vi "myRIO v1.0 Build Bitmask DIO.vi"(10 "bool Value List In":bool[](array[boolean]), 11 "Channel List":T3) -> (1 "Bitmask to Channel Array":T1[](array[typedef]), 2 "OUT Bitmask Array":bool[][](array[boolean]), 3 "DIR Bitmask Array":bool[][](array[boolean]))   [LabVIEW 2021]
uses:
  <vilib>/myRIO/Common/Instrument Driver Framework/myRIO v1.0/DIO/typedefs/DIO Channels List.ctl
  <vilib>/myRIO/Common/Instrument Driver Framework/myRIO v1.0/DIO/typedefs/DIO Channels Enum.ctl
  <vilib>/myRIO/Common/Instrument Driver Framework/myRIO v1.0/DIO/typedefs/DIO Bitmask to Channel Map.ctl
  <vilib>/myRIO/Common/Instrument Driver Framework/myRIO v1.0/DIO/typedefs/DIO Bank Enum.ctl
panel:
  # "This VI is used by both the myRIO v1.0 Read DIO and Write DIO VIs. \nIf a bool Value List in is provided the appropriate OUT Botmask Array will be generated, otherwise all values in the array will be false."
  # "*Only Used for DIO Write"
  # "*Only Used for DIO Write"
  # "*Only Used for DIO Read"
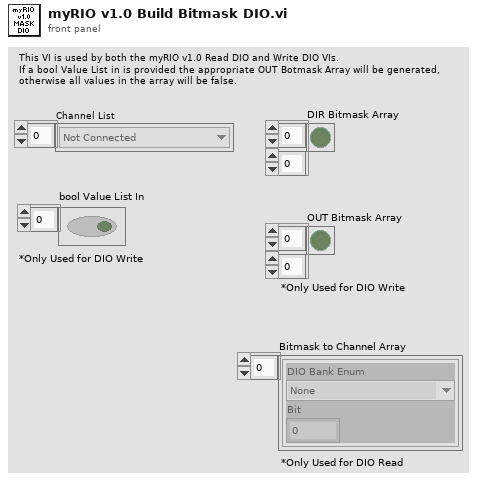
[diagram p1: front panel]
types:
  T1 = typedef "DIO Bitmask to Channel Map.ctl" = cluster{"DIO Bank Enum":T2, "Bit":i32}
  T2 = typedef "DIO Bank Enum.ctl" = enum32{"None", "C/DIO7:0", "A/DIO7:0", "A/DIO15:8", "B/DIO7:0", "B/DIO15:8", "LED3:0", "Button0"}
  T3 = typedef "DIO Channels List.ctl" = T4[]
  T4 = typedef "DIO Channels Enum.ctl" = enum16{"Not Connected", "C/DIO0", "C/DIO1", "C/DIO2", "C/DIO3", "C/DIO4", "C/DIO5", "C/DIO6", "C/DIO7", "A/DIO0", "A/DIO1", "A/DIO2", "A/DIO3", "A/DIO4", "A/DIO5", "A/DIO6", "A/DIO7", "A/DIO8", "A/DIO9", "A/DIO10", "A/DIO11", "A/DIO12", "A/DIO13", "A/DIO14", "A/DIO15", "A/DIO16", "A/DIO17", "A/DIO18", "A/DIO19", "B/DIO0", "B/DIO1", "B/DIO2", "B/DIO3", "B/DIO4", "B/DIO5", "B/DIO6", "B/DIO7", "B/DIO8", "B/DIO9", "B/DIO10", "B/DIO11", "B/DIO12", "B/DIO13", "B/DIO14", "B/DIO15", "B/DIO16", "B/DIO17", "B/DIO18", "B/DIO19", "LED0", "LED1", "LED2", "LED3", "Button0", "DIO/DIO0", "DIO/DIO1", "DIO/DIO2", "DIO/DIO3", "DIO/DIO4", "DIO/DIO5", "DIO/DIO6", "DIO/DIO7", "DIO/DIO8", "DIO/DIO9", "SPI/CS0", "SPI/CS1", "SPI/CS2", "SPI/CS3", "LED RADIO (Green)", "LED RADIO (Red)", "LED COMM (Green)", "LED COMM (Red)", "LED MODE (Green)", "LED MODE (Red)"}
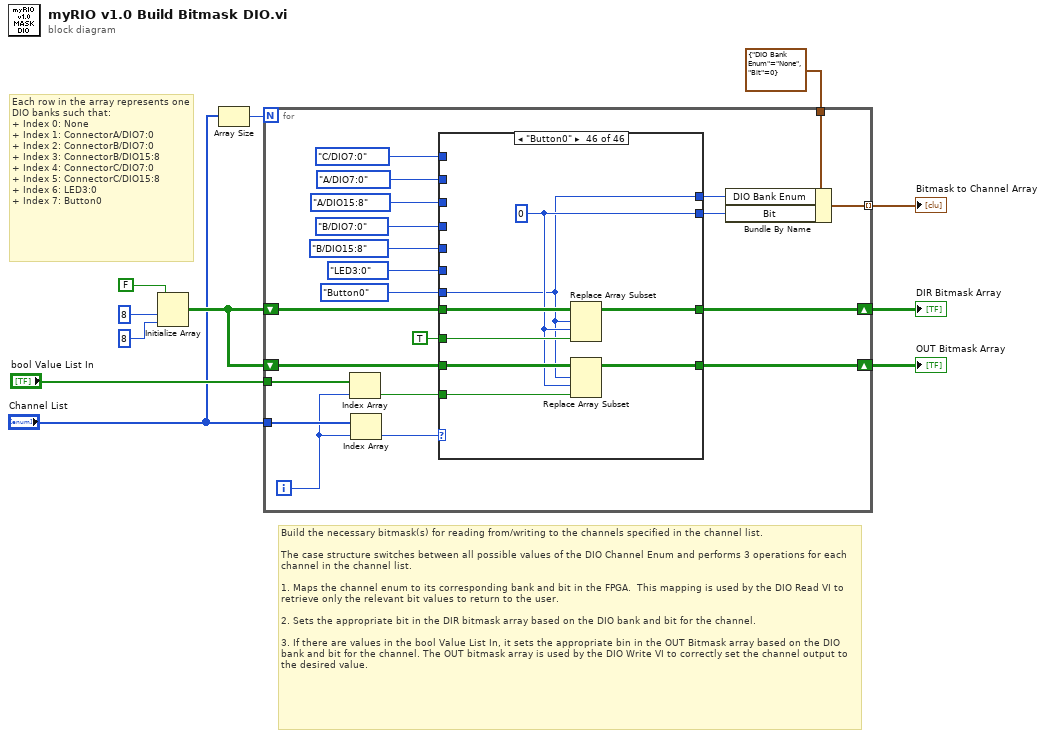
[diagram p0: block diagram]
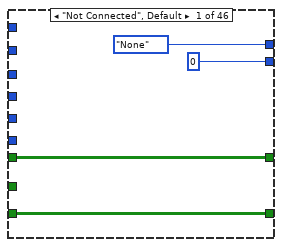
[diagram p2: hidden frame]
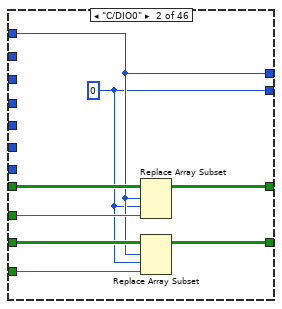
[diagram p3: hidden frame]
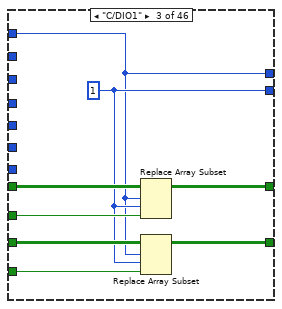
[diagram p4: hidden frame]
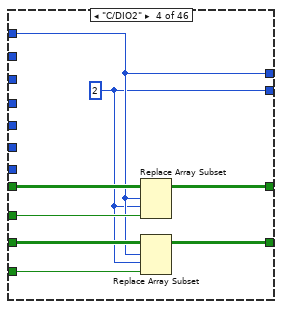
[diagram p5: hidden frame]
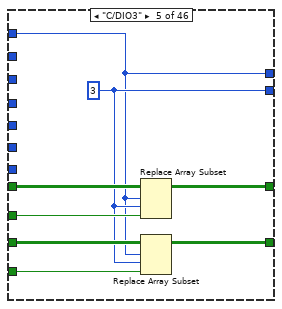
[diagram p6: hidden frame]
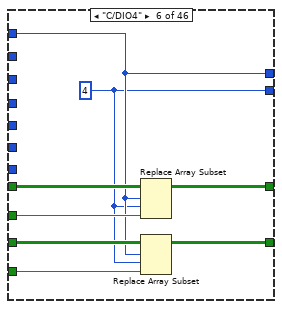
[diagram p7: hidden frame]
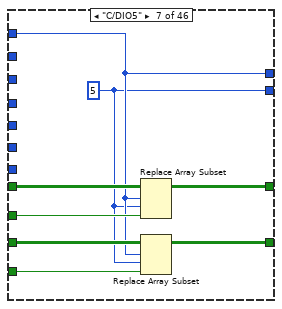
[diagram p8: hidden frame]
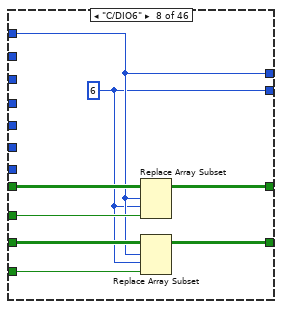
[diagram p9: hidden frame]
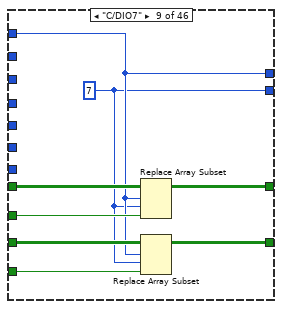
[diagram p10: hidden frame]
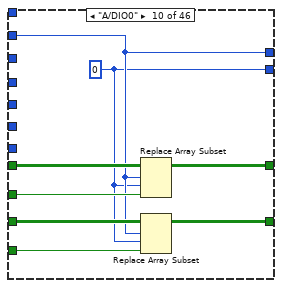
[diagram p11: hidden frame]
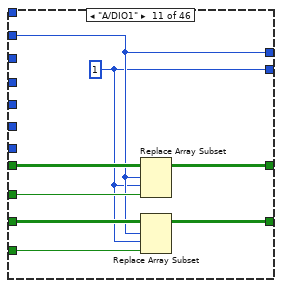
[diagram p12: hidden frame]
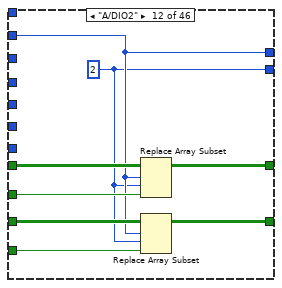
[diagram p13: hidden frame]
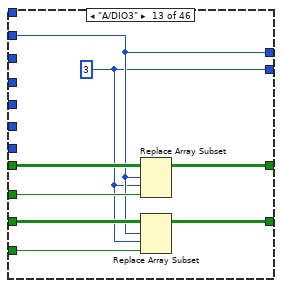
[diagram p14: hidden frame]
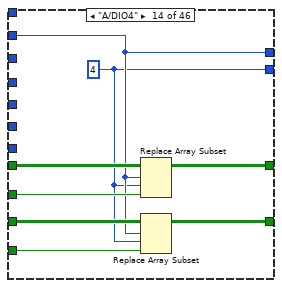
[diagram p15: hidden frame]
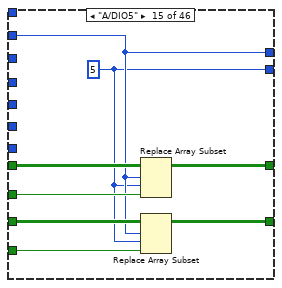
[diagram p16: hidden frame]
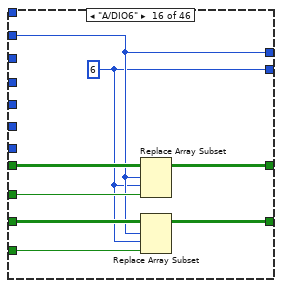
[diagram p17: hidden frame]
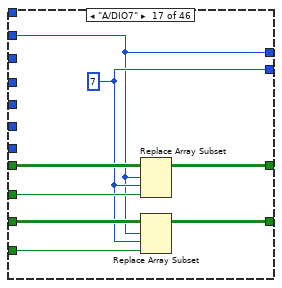
[diagram p18: hidden frame]
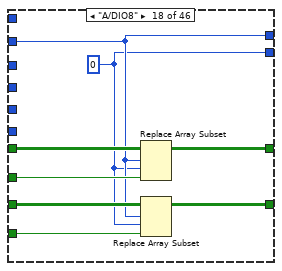
[diagram p19: hidden frame]
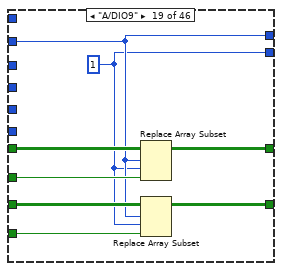
[diagram p20: hidden frame]
diagram:
  # "Build the necessary bitmask(s) for reading from/writing to the channels specified in the channel list.\n\nThe case structure switches between all possible values of the DIO Channel Enum and performs 3 operations for each channel in the channel list. \n\n1. Maps the channel enum to its corresponding bank and bit in the FPGA.  This mapping is used by the DIO Read VI to retrieve only the relevant bit values to return to the user.\n\n2. Sets the appropriate bit in the DIR bitmask array based on the DIO bank and bit for the channel.\n\n3. If there are values in the bool Value List In, it sets the appropriate bin in the OUT Bitmask array based on the DIO bank and bit for the channel. The OUT bitmask array is used by the DIO Write VI to correctly set the channel output to the desired value."
  # "Each row in the array represents one DIO banks such that:\n+ Index 0: None\n+ Index 1: ConnectorA/DIO7:0\n+ Index 2: ConnectorB/DIO7:0\n+ Index 3: ConnectorB/DIO15:8\n+ Index 4: ConnectorC/DIO7:0\n+ Index 5: ConnectorC/DIO15:8\n+ Index 6: LED3:0\n+ Index 7: Button0"
  n1 = Initialize Array(FALSE, 8 ("dimension size"), 8 ("dimension size")) -> (w5:bool[][])
  n2 = Array Size(array="Channel List") -> (size(s)=w2:i32)
  n3 = for {
    N: w2 -> [_]
    tunnel: "Channel List" -> [w17]
    shift-right: [w30] -> w10
    shift-left: w5 -> [w32]
    tunnel: T1 {"DIO Bank Enum"=enum."None", "Bit"=0} -> [w29]
    tunnel: [w27] -> w6 mode=indexing
    shift-right: [w19] -> w4
    shift-left: w5 -> [w20]
    tunnel: "bool Value List In" -> [w18]
    i -> [w15]
    n4 = Index Array(array=w18, index=w15) -> (element=w14:bool)
    n5 = Index Array(array=w17, index=w15) -> (element=w16:T4)
    n6 = case shown="\"Button0\"" w16 {
      tunnel: w32 -> [w36 w44 w52 w60 w68 w76 w84 w92 w100 w108 w116 w124 w132 w140 w148 w156 w164 w172 w180 w188 w196 w204 w212 w220 w228 w236 w244 w252 w260 w268 w276 w284 w292 w300 w308 w316 w324 w332 w340 w348 w356 w364 w372 w380 w388 w396]
      tunnel: TRUE ("new element/subarray") -> [_ w42 w50 w59 w67 w74 w82 w90 w99 w107 w114 w123 w130 w138 w146 w154 w162 w170 w178 w186 w194 w202 w210 w218 w226 w234 w242 w250 w258 w266 w274 w282 w290 w298 w306 w314 w322 w330 w338 w346 w355 w363 w371 w379 w387 w395]
      tunnel: [w36 w43 w51 w58 w66 w75 w83 w91 w98 w106 w115 w121 w131 w139 w147 w155 w163 w171 w179 w187 w195 w203 w211 w219 w227 w235 w243 w251 w259 w267 w275 w283 w291 w299 w307 w315 w323 w331 w339 w347 w354 w362 w370 w378 w386 w394] -> w30
      tunnel: [0 ("disabled index (col)") w38 w47 w54 w63 w70 w78 w86 w94 w102 w110 w118 w125 w134 w142 w150 w159 w166 w174 w182 w190 w198 w206 w214 w222 w231 w239 w247 w255 w263 w271 w279 w287 w295 w303 w311 w319 w327 w335 w343 w350 w359 w367 w375 w383 w391] -> w28
      tunnel: [DIO_Bank_Enum."None" ("DIO Bank Enum") w39 w46 w55 w62 w71 w79 w87 w95 w103 w111 w119 w126 w135 w143 w151 w157 w167 w175 w183 w191 w199 w207 w215 w223 w229 w237 w245 w253 w261 w269 w277 w285 w293 w301 w309 w317 w325 w333 w341 w351 w357 w365 w373 w381 w389] -> w25
      tunnel: DIO_Bank_Enum."C/DIO7:0" ("DIO Bank Enum") -> [_ w39 w46 w55 w62 w71 w79 w87 w95 _ _ _ _ _ _ _ _ _ _ _ _ _ _ _ _ _ _ _ _ _ _ _ _ _ _ _ _ _ _ _ _ _ _ _ _ _]
      tunnel: DIO_Bank_Enum."A/DIO7:0" ("DIO Bank Enum") -> [_ _ _ _ _ _ _ _ _ w103 w111 w119 w126 w135 w143 w151 w157 _ _ _ _ _ _ _ _ _ _ _ _ _ _ _ _ _ _ _ _ _ _ _ _ _ _ _ _ _]
      tunnel: DIO_Bank_Enum."A/DIO15:8" ("DIO Bank Enum") -> [_ _ _ _ _ _ _ _ _ _ _ _ _ _ _ _ _ w167 w175 w183 w191 w199 w207 w215 w223 _ _ _ _ _ _ _ _ _ _ _ _ _ _ _ _ _ _ _ _ _]
      tunnel: DIO_Bank_Enum."B/DIO7:0" ("DIO Bank Enum") -> [_ _ _ _ _ _ _ _ _ _ _ _ _ _ _ _ _ _ _ _ _ _ _ _ _ w229 w237 w245 w253 w261 w269 w277 w285 _ _ _ _ _ _ _ _ _ _ _ _ _]
      tunnel: DIO_Bank_Enum."B/DIO15:8" ("DIO Bank Enum") -> [_ _ _ _ _ _ _ _ _ _ _ _ _ _ _ _ _ _ _ _ _ _ _ _ _ _ _ _ _ _ _ _ _ w293 w301 w309 w317 w325 w333 w341 w351 _ _ _ _ _]
      tunnel: w20 -> [w33 w41 w49 w57 w65 w73 w81 w89 w97 w104 w112 w122 w129 w137 w144 w152 w160 w168 w176 w184 w192 w200 w208 w216 w224 w232 w240 w248 w256 w264 w272 w280 w288 w296 w304 w312 w320 w328 w336 w344 w353 w361 w369 w377 w385 w393]
      tunnel: [w33 w40 w48 w56 w64 w72 w80 w88 w96 w105 w113 w120 w128 w136 w145 w153 w161 w169 w177 w185 w193 w201 w209 w217 w225 w233 w241 w249 w257 w265 w273 w281 w289 w297 w305 w313 w321 w329 w337 w345 w352 w360 w368 w376 w384 w392] -> w19
      tunnel: w14 -> [_ w37 w45 w53 w61 w69 w77 w85 w93 w101 w109 w117 w127 w133 w141 w149 w158 w165 w173 w181 w189 w197 w205 w213 w221 w230 w238 w246 w254 w262 w270 w278 w286 w294 w302 w310 w318 w326 w334 w342 w349 w358 w366 w374 w382 w390]
      tunnel: DIO_Bank_Enum."LED3:0" ("DIO Bank Enum") -> [_ _ _ _ _ _ _ _ _ _ _ _ _ _ _ _ _ _ _ _ _ _ _ _ _ _ _ _ _ _ _ _ _ _ _ _ _ _ _ _ _ w357 w365 w373 w381 _]
      tunnel: DIO_Bank_Enum."Button0" ("DIO Bank Enum") -> [_ _ _ _ _ _ _ _ _ _ _ _ _ _ _ _ _ _ _ _ _ _ _ _ _ _ _ _ _ _ _ _ _ _ _ _ _ _ _ _ _ _ _ _ _ w389]
      frame "Not Connected", Default {
      }
      frame "C/DIO0" {
        w38 = 0 ("disabled index (col)")
        n7 = Replace Array Subset(array=w44, new element=w42, index (row)=w39, index (col)=w38) -> (w43:bool[][])
        n8 = Replace Array Subset(array=w41, new element=w37, index (row)=w39, index (col)=w38) -> (w40:bool[][])
      }
      frame "C/DIO1" {
        w47 = 1 ("disabled index (col)")
        n9 = Replace Array Subset(array=w52, new element=w50, index (row)=w46, index (col)=w47) -> (w51:bool[][])
        n10 = Replace Array Subset(array=w49, new element=w45, index (row)=w46, index (col)=w47) -> (w48:bool[][])
      }
      frame "C/DIO2" {
        w54 = 2 ("disabled index (col)")
        n11 = Replace Array Subset(array=w60, new element=w59, index (row)=w55, index (col)=w54) -> (w58:bool[][])
        n12 = Replace Array Subset(array=w57, new element=w53, index (row)=w55, index (col)=w54) -> (w56:bool[][])
      }
      frame "C/DIO3" {
        w63 = 3 ("disabled index (col)")
        n13 = Replace Array Subset(array=w68, new element=w67, index (row)=w62, index (col)=w63) -> (w66:bool[][])
        n14 = Replace Array Subset(array=w65, new element=w61, index (row)=w62, index (col)=w63) -> (w64:bool[][])
      }
      frame "C/DIO4" {
        w70 = 4 ("disabled index (col)")
        n15 = Replace Array Subset(array=w76, new element=w74, index (row)=w71, index (col)=w70) -> (w75:bool[][])
        n16 = Replace Array Subset(array=w73, new element=w69, index (row)=w71, index (col)=w70) -> (w72:bool[][])
      }
      frame "C/DIO5" {
        w78 = 5 ("disabled index (col)")
        n17 = Replace Array Subset(array=w84, new element=w82, index (row)=w79, index (col)=w78) -> (w83:bool[][])
        n18 = Replace Array Subset(array=w81, new element=w77, index (row)=w79, index (col)=w78) -> (w80:bool[][])
      }
      frame "C/DIO6" {
        w86 = 6 ("disabled index (col)")
        n19 = Replace Array Subset(array=w92, new element=w90, index (row)=w87, index (col)=w86) -> (w91:bool[][])
        n20 = Replace Array Subset(array=w89, new element=w85, index (row)=w87, index (col)=w86) -> (w88:bool[][])
      }
      frame "C/DIO7" {
        w94 = 7 ("disabled index (col)")
        n21 = Replace Array Subset(array=w100, new element=w99, index (row)=w95, index (col)=w94) -> (w98:bool[][])
        n22 = Replace Array Subset(array=w97, new element=w93, index (row)=w95, index (col)=w94) -> (w96:bool[][])
      }
      frame "A/DIO0" {
        w102 = 0 ("disabled index (col)")
        n23 = Replace Array Subset(array=w108, new element=w107, index (row)=w103, index (col)=w102) -> (w106:bool[][])
        n24 = Replace Array Subset(array=w104, new element=w101, index (row)=w103, index (col)=w102) -> (w105:bool[][])
      }
      frame "A/DIO1" {
        w110 = 1 ("disabled index (col)")
        n25 = Replace Array Subset(array=w116, new element=w114, index (row)=w111, index (col)=w110) -> (w115:bool[][])
        n26 = Replace Array Subset(array=w112, new element=w109, index (row)=w111, index (col)=w110) -> (w113:bool[][])
      }
      frame "A/DIO2" {
        w118 = 2 ("disabled index (col)")
        n27 = Replace Array Subset(array=w124, new element=w123, index (row)=w119, index (col)=w118) -> (w121:bool[][])
        n28 = Replace Array Subset(array=w122, new element=w117, index (row)=w119, index (col)=w118) -> (w120:bool[][])
      }
      frame "A/DIO3" {
        w125 = 3 ("disabled index (col)")
        n29 = Replace Array Subset(array=w132, new element=w130, index (row)=w126, index (col)=w125) -> (w131:bool[][])
        n30 = Replace Array Subset(array=w129, new element=w127, index (row)=w126, index (col)=w125) -> (w128:bool[][])
      }
      frame "A/DIO4" {
        w134 = 4 ("disabled index (col)")
        n31 = Replace Array Subset(array=w140, new element=w138, index (row)=w135, index (col)=w134) -> (w139:bool[][])
        n32 = Replace Array Subset(array=w137, new element=w133, index (row)=w135, index (col)=w134) -> (w136:bool[][])
      }
      frame "A/DIO5" {
        w142 = 5 ("disabled index (col)")
        n33 = Replace Array Subset(array=w148, new element=w146, index (row)=w143, index (col)=w142) -> (w147:bool[][])
        n34 = Replace Array Subset(array=w144, new element=w141, index (row)=w143, index (col)=w142) -> (w145:bool[][])
      }
      frame "A/DIO6" {
        w150 = 6 ("disabled index (col)")
        n35 = Replace Array Subset(array=w156, new element=w154, index (row)=w151, index (col)=w150) -> (w155:bool[][])
        n36 = Replace Array Subset(array=w152, new element=w149, index (row)=w151, index (col)=w150) -> (w153:bool[][])
      }
      frame "A/DIO7" {
        w159 = 7 ("disabled index (col)")
        n37 = Replace Array Subset(array=w164, new element=w162, index (row)=w157, index (col)=w159) -> (w163:bool[][])
        n38 = Replace Array Subset(array=w160, new element=w158, index (row)=w157, index (col)=w159) -> (w161:bool[][])
      }
      frame "A/DIO8" {
        w166 = 0 ("disabled index (col)")
        n39 = Replace Array Subset(array=w172, new element=w170, index (row)=w167, index (col)=w166) -> (w171:bool[][])
        n40 = Replace Array Subset(array=w168, new element=w165, index (row)=w167, index (col)=w166) -> (w169:bool[][])
      }
      frame "A/DIO9" {
        w174 = 1 ("disabled index (col)")
        n41 = Replace Array Subset(array=w180, new element=w178, index (row)=w175, index (col)=w174) -> (w179:bool[][])
        n42 = Replace Array Subset(array=w176, new element=w173, index (row)=w175, index (col)=w174) -> (w177:bool[][])
      }
      frame "A/DIO10" {
        w182 = 2 ("disabled index (col)")
        n43 = Replace Array Subset(array=w188, new element=w186, index (row)=w183, index (col)=w182) -> (w187:bool[][])
        n44 = Replace Array Subset(array=w184, new element=w181, index (row)=w183, index (col)=w182) -> (w185:bool[][])
      }
      frame "A/DIO11" {
        w190 = 3 ("disabled index (col)")
        n45 = Replace Array Subset(array=w196, new element=w194, index (row)=w191, index (col)=w190) -> (w195:bool[][])
        n46 = Replace Array Subset(array=w192, new element=w189, index (row)=w191, index (col)=w190) -> (w193:bool[][])
      }
      frame "A/DIO12" {
        w198 = 4 ("disabled index (col)")
        n47 = Replace Array Subset(array=w204, new element=w202, index (row)=w199, index (col)=w198) -> (w203:bool[][])
        n48 = Replace Array Subset(array=w200, new element=w197, index (row)=w199, index (col)=w198) -> (w201:bool[][])
      }
      frame "A/DIO13" {
        w206 = 5 ("disabled index (col)")
        n49 = Replace Array Subset(array=w212, new element=w210, index (row)=w207, index (col)=w206) -> (w211:bool[][])
        n50 = Replace Array Subset(array=w208, new element=w205, index (row)=w207, index (col)=w206) -> (w209:bool[][])
      }
      frame "A/DIO14" {
        w214 = 6 ("disabled index (col)")
        n51 = Replace Array Subset(array=w220, new element=w218, index (row)=w215, index (col)=w214) -> (w219:bool[][])
        n52 = Replace Array Subset(array=w216, new element=w213, index (row)=w215, index (col)=w214) -> (w217:bool[][])
      }
      frame "A/DIO15" {
        w222 = 7 ("disabled index (col)")
        n53 = Replace Array Subset(array=w228, new element=w226, index (row)=w223, index (col)=w222) -> (w227:bool[][])
        n54 = Replace Array Subset(array=w224, new element=w221, index (row)=w223, index (col)=w222) -> (w225:bool[][])
      }
      frame "B/DIO0" {
        w231 = 0 ("disabled index (col)")
        n55 = Replace Array Subset(array=w236, new element=w234, index (row)=w229, index (col)=w231) -> (w235:bool[][])
        n56 = Replace Array Subset(array=w232, new element=w230, index (row)=w229, index (col)=w231) -> (w233:bool[][])
      }
      frame "B/DIO1" {
        w239 = 1 ("disabled index (col)")
        n57 = Replace Array Subset(array=w244, new element=w242, index (row)=w237, index (col)=w239) -> (w243:bool[][])
        n58 = Replace Array Subset(array=w240, new element=w238, index (row)=w237, index (col)=w239) -> (w241:bool[][])
      }
      frame "B/DIO2" {
        w247 = 2 ("disabled index (col)")
        n59 = Replace Array Subset(array=w252, new element=w250, index (row)=w245, index (col)=w247) -> (w251:bool[][])
        n60 = Replace Array Subset(array=w248, new element=w246, index (row)=w245, index (col)=w247) -> (w249:bool[][])
      }
      frame "B/DIO3" {
        w255 = 3 ("disabled index (col)")
        n61 = Replace Array Subset(array=w260, new element=w258, index (row)=w253, index (col)=w255) -> (w259:bool[][])
        n62 = Replace Array Subset(array=w256, new element=w254, index (row)=w253, index (col)=w255) -> (w257:bool[][])
      }
      frame "B/DIO4" {
        w263 = 4 ("disabled index (col)")
        n63 = Replace Array Subset(array=w268, new element=w266, index (row)=w261, index (col)=w263) -> (w267:bool[][])
        n64 = Replace Array Subset(array=w264, new element=w262, index (row)=w261, index (col)=w263) -> (w265:bool[][])
      }
      frame "B/DIO5" {
        w271 = 5 ("disabled index (col)")
        n65 = Replace Array Subset(array=w276, new element=w274, index (row)=w269, index (col)=w271) -> (w275:bool[][])
        n66 = Replace Array Subset(array=w272, new element=w270, index (row)=w269, index (col)=w271) -> (w273:bool[][])
      }
      frame "B/DIO6" {
        w279 = 6 ("disabled index (col)")
        n67 = Replace Array Subset(array=w284, new element=w282, index (row)=w277, index (col)=w279) -> (w283:bool[][])
        n68 = Replace Array Subset(array=w280, new element=w278, index (row)=w277, index (col)=w279) -> (w281:bool[][])
      }
      frame "B/DIO7" {
        w287 = 7 ("disabled index (col)")
        n69 = Replace Array Subset(array=w292, new element=w290, index (row)=w285, index (col)=w287) -> (w291:bool[][])
        n70 = Replace Array Subset(array=w288, new element=w286, index (row)=w285, index (col)=w287) -> (w289:bool[][])
      }
      frame "B/DIO8" {
        w295 = 0 ("disabled index (col)")
        n71 = Replace Array Subset(array=w300, new element=w298, index (row)=w293, index (col)=w295) -> (w299:bool[][])
        n72 = Replace Array Subset(array=w296, new element=w294, index (row)=w293, index (col)=w295) -> (w297:bool[][])
      }
      frame "B/DIO9" {
        w303 = 1 ("disabled index (col)")
        n73 = Replace Array Subset(array=w308, new element=w306, index (row)=w301, index (col)=w303) -> (w307:bool[][])
        n74 = Replace Array Subset(array=w304, new element=w302, index (row)=w301, index (col)=w303) -> (w305:bool[][])
      }
      frame "B/DIO10" {
        w311 = 2 ("disabled index (col)")
        n75 = Replace Array Subset(array=w316, new element=w314, index (row)=w309, index (col)=w311) -> (w315:bool[][])
        n76 = Replace Array Subset(array=w312, new element=w310, index (row)=w309, index (col)=w311) -> (w313:bool[][])
      }
      frame "B/DIO11" {
        w319 = 3 ("disabled index (col)")
        n77 = Replace Array Subset(array=w324, new element=w322, index (row)=w317, index (col)=w319) -> (w323:bool[][])
        n78 = Replace Array Subset(array=w320, new element=w318, index (row)=w317, index (col)=w319) -> (w321:bool[][])
      }
      frame "B/DIO12" {
        w327 = 4 ("disabled index (col)")
        n79 = Replace Array Subset(array=w332, new element=w330, index (row)=w325, index (col)=w327) -> (w331:bool[][])
        n80 = Replace Array Subset(array=w328, new element=w326, index (row)=w325, index (col)=w327) -> (w329:bool[][])
      }
      frame "B/DIO13" {
        w335 = 5 ("disabled index (col)")
        n81 = Replace Array Subset(array=w340, new element=w338, index (row)=w333, index (col)=w335) -> (w339:bool[][])
        n82 = Replace Array Subset(array=w336, new element=w334, index (row)=w333, index (col)=w335) -> (w337:bool[][])
      }
      frame "B/DIO14" {
        w343 = 6 ("disabled index (col)")
        n83 = Replace Array Subset(array=w348, new element=w346, index (row)=w341, index (col)=w343) -> (w347:bool[][])
        n84 = Replace Array Subset(array=w344, new element=w342, index (row)=w341, index (col)=w343) -> (w345:bool[][])
      }
      frame "B/DIO15" {
        w350 = 7 ("disabled index (col)")
        n85 = Replace Array Subset(array=w356, new element=w355, index (row)=w351, index (col)=w350) -> (w354:bool[][])
        n86 = Replace Array Subset(array=w353, new element=w349, index (row)=w351, index (col)=w350) -> (w352:bool[][])
      }
      frame "LED0" {
        w359 = 0 ("disabled index (col)")
        n87 = Replace Array Subset(array=w364, new element=w363, index (row)=w357, index (col)=w359) -> (w362:bool[][])
        n88 = Replace Array Subset(array=w361, new element=w358, index (row)=w357, index (col)=w359) -> (w360:bool[][])
      }
      frame "LED1" {
        w367 = 1 ("disabled index (col)")
        n89 = Replace Array Subset(array=w372, new element=w371, index (row)=w365, index (col)=w367) -> (w370:bool[][])
        n90 = Replace Array Subset(array=w369, new element=w366, index (row)=w365, index (col)=w367) -> (w368:bool[][])
      }
      frame "LED2" {
        w375 = 2 ("disabled index (col)")
        n91 = Replace Array Subset(array=w380, new element=w379, index (row)=w373, index (col)=w375) -> (w378:bool[][])
        n92 = Replace Array Subset(array=w377, new element=w374, index (row)=w373, index (col)=w375) -> (w376:bool[][])
      }
      frame "LED3" {
        w383 = 3 ("disabled index (col)")
        n93 = Replace Array Subset(array=w388, new element=w387, index (row)=w381, index (col)=w383) -> (w386:bool[][])
        n94 = Replace Array Subset(array=w385, new element=w382, index (row)=w381, index (col)=w383) -> (w384:bool[][])
      }
      frame "Button0" {
        w391 = 0 ("disabled index (col)")
        n95 = Replace Array Subset(array=w396, new element=w395, index (row)=w389, index (col)=w391) -> (w394:bool[][])
        n96 = Replace Array Subset(array=w393, new element=w390, index (row)=w389, index (col)=w391) -> (w392:bool[][])
      }
    }
    n97 = Bundle By Name(cluster=w29, "DIO Bank Enum"=w25, "Bit"=w28) -> (w27:T1)
  }
  "DIR Bitmask Array" <- w10
  "Bitmask to Channel Array" <- w6
  "OUT Bitmask Array" <- w4
